vi "测试.vi"() -> ()   [LabVIEW 2016]
panel:
  in  "选择类名称 2":u16(ring) items=["黑糯米奶茶", "招牌奶茶", "茉莉奶茶"]
  in  "数组":refnum<class "醇香奶茶.lvclass">[](array[class])
  in  "选择类名称":u16(ring) items=["黑糯米奶茶", "招牌奶茶", "茉莉奶茶"]
  out "价格":dbl
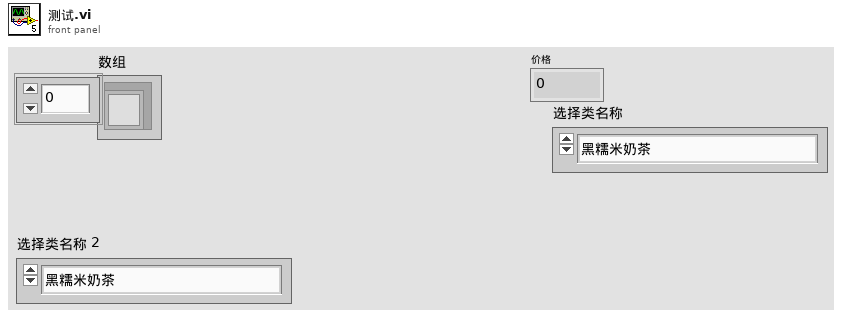
[diagram p1: front panel]
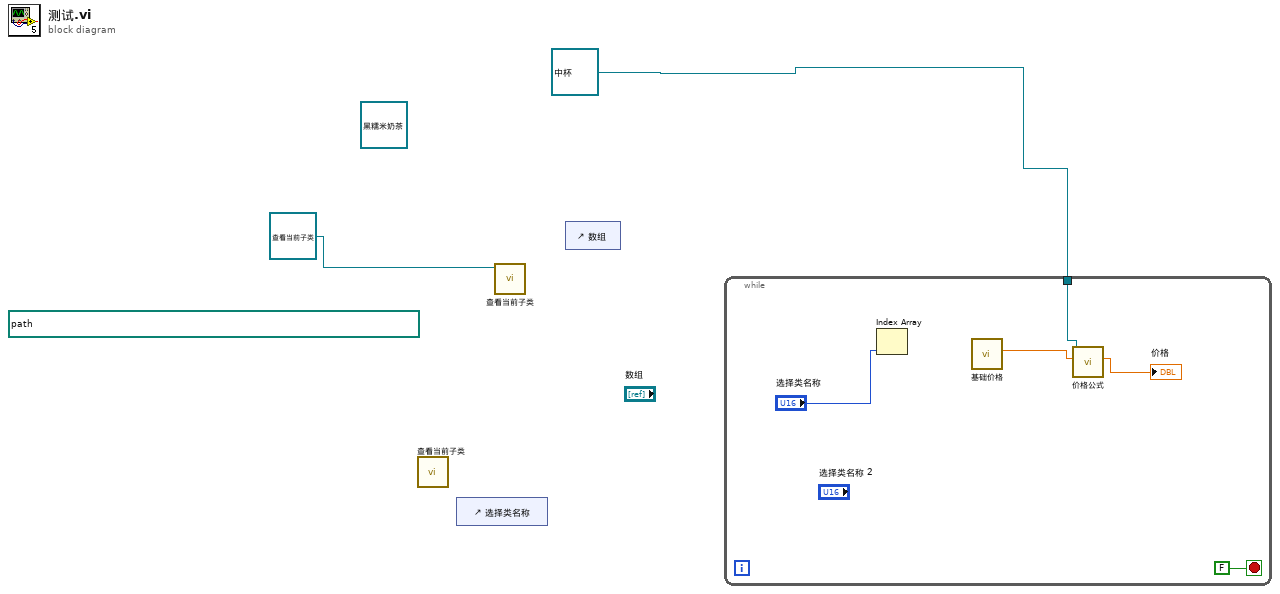
[diagram p0: block diagram]
diagram:
  (unwired) path "C:/Users/lenovo/Desktop/奶茶店/奶茶/醇香奶茶" ("Folder Path")
  (unwired) refnum<class "黑糯米奶茶.lvclass"> refnum ("黑糯米奶茶.lvclass")
  n1 = call-dynamic "查看当前子类.vi"() -> ()  [unwired: 8 in, 4 out]
  n2 = control-ref of="选择类名称"() -> ()  [unwired: 1 out]
  n3 = call-dynamic "查看当前子类.vi"("查看当前子类 输入"=refnum<class "查看当前子类.lvclass"> refnum ("查看当前子类.lvclass")) -> ()  [unwired: 7 in, 4 out]
  n4 = control-ref of="数组"() -> ()  [unwired: 1 out]
  n5 = while {
    tunnel: refnum<class "中杯.lvclass"> refnum ("中杯.lvclass") -> [w5]
    stop <- FALSE stop-if-true
    n6 = Index Array(index="选择类名称") -> ()  [unwired: 1 in, 1 out]
    n7 = call-dynamic "基础价格.vi"() -> ("基础价格"=w6:dbl)  [unwired: 9 in, 2 out]
    n8 = call-dynamic "价格公式.vi"("基础价格"=w6, "中杯 输入"=w5) -> ("价格"=→"价格":dbl)  [unwired: 7 in, 2 out]
  }
